vi "题目2.vi"() -> ()   [LabVIEW 2017]
panel:
  out "数值 2":i32
  out "数值":dbl
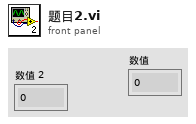
[diagram p1: front panel]
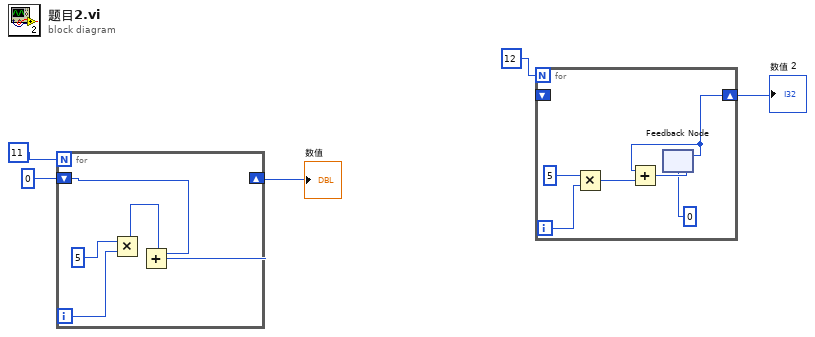
[diagram p0: block diagram]
diagram:
  n1 = for {
    N: 11 -> [_]
    shift-right: [w9] -> w2
    shift-left: 0 -> [w6]
    i -> [w10]
    n2 = Multiply(x=5, y=w10) -> (x*y=w7:i32)
    n3 = Add(x=w6, y=w7) -> (x+y=w9:i32)
  }
  "数值" <- w2
  n4 = for {
    N: 12 -> [_]
    shift-right: [w11] -> w1
    shift-left: _ -> [_]
    i -> [w15]
    n5 = Multiply(x=5, y=w15) -> (x*y=w14:i32)
    n6 = feedback #1(0) -> (w11:i32)
    n7 = Add(x=w11, y=w14) -> (x+y=w13:i32)
    n8 = feedback-in #1(w13) -> ()
  }
  "数值 2" <- w1
